vi "실습 2.vi"() -> ()   [LabVIEW 2014]
uses:
  <vilib>/Analysis/NI_AALBase.lvlib
panel:
  out "웨이브폼 그래프":dbl[](graph)
  in  "Task":bool
  in  "정지":bool
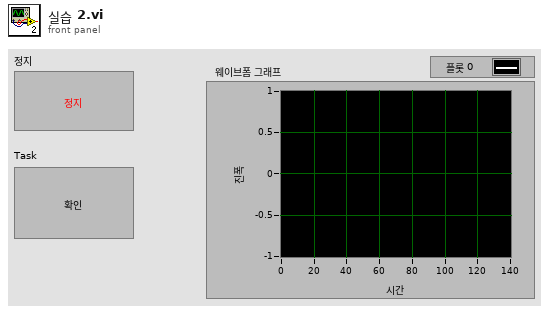
[diagram p1: front panel]
types:
  T1 = typedef "상태.ctl" = enum16{"Idle", "초기화", "Stop", "task01", "task02", "2초 기다림 ", "Task03"}
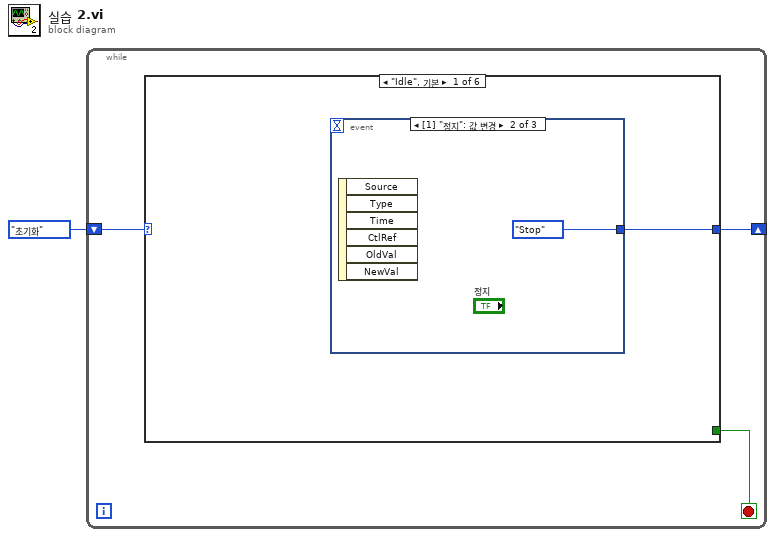
[diagram p0: block diagram]
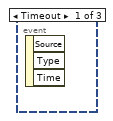
[diagram p2: hidden frame]
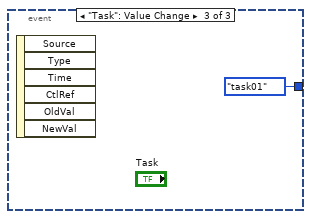
[diagram p3: hidden frame]
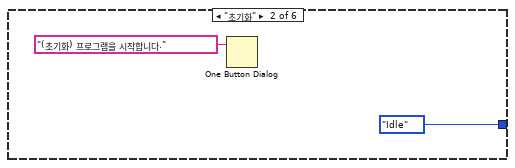
[diagram p4: hidden frame]
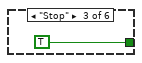
[diagram p5: hidden frame]
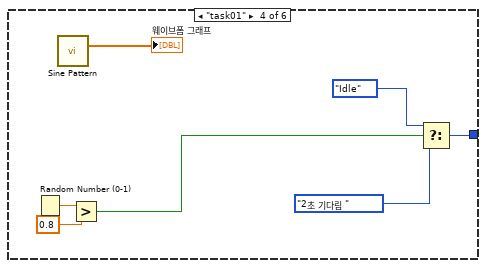
[diagram p6: hidden frame]
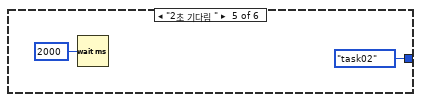
[diagram p7: hidden frame]
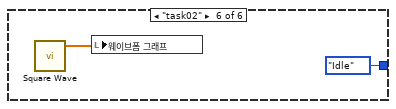
[diagram p8: hidden frame]
diagram:
  n1 = while {
    shift-right: [w3] -> _
    shift-left: 상태."초기화" -> [w4]
    stop <- w2 stop-if-true
    n2 = case shown="\"Idle\", 기본" w4 {
      tunnel: [w5 상태."Idle" _ w14 상태."task02" 상태."Idle"] -> w3
      tunnel: [_ _ TRUE _ _ _] -> w2
      frame "Idle", Default {
        n3 = event shown="[1] \"정지\": 값 변경" {
          selector: _ -> [_ _ _]
          dyn-events: _ -> [_ _ _]
          timeout: _ -> [_ _ _]
          tunnel: [_ 상태."Stop" 상태."task01"] -> w5
          event Timeout {
            n4 = event-data() -> ()  [unwired: 1 in, 3 out]
          }
          event "정지": Value Change {
            n5 = event-data() -> ()  [unwired: 1 in, 6 out]
          }
          event "Task": Value Change {
            n6 = event-data() -> ()  [unwired: 1 in, 6 out]
          }
        }
      }
      frame "초기화" {
        n7 = One Button Dialog(message="(초기화) 프로그램을 시작합니다." ("메시지")) -> ()  [unwired: 1 in, 1 out]
      }
      frame "Stop" {
      }
      frame "task01" {
        n8 = Random Number (0-1)() -> (number: 0 to 1=w13:dbl)
        n9 = call <vilib>:"Sine Pattern.vi"() -> ("Sinusoidal Pattern"=→"웨이브폼 그래프":dbl[])  [unwired: 4 in, 1 out]
        n10 = Greater?(x=w13, y=0.8) -> (0:w11:bool)
        n11 = Select(t=상태."Idle", s=w11, f=상태."2초 기다림 ") -> (s? t:f=w14:T1)
      }
      frame "2초 기다림 " {
        n12 = Wait (ms)(milliseconds to wait=u32 2000 ("대기 시간(ms)")) -> ()  [unwired: 1 out]
      }
      frame "task02" {
        n13 = call <vilib>:"Square Wave.vi"() -> ("square wave"=w20:dbl[])  [unwired: 6 in, 2 out]
        n14 = local write "웨이브폼 그래프"(w20) -> ()
      }
    }
  }
